vi "from string.vi"(8 "error in":errorcluster, 9 "data":string, 10 "version":string, 11 "Engine configuration in":refnum<class "Engine configuration.lvclass">) -> (0 "error out":errorcluster, 3 "Engine configuration out":refnum<class "Engine configuration.lvclass">)   [LabVIEW 2025, in "Abstract Engine.lvlib" / "Engine configuration.lvclass"]
doc: "Provides an interface for loading a module configuration from a file or other serialized data source. It is recommended that all children of this class store data in two sets--data required for its own initialization, and any data required for parent initialization--and that each implementation uses the <b>Call Parent Method</b> primitive to de-serialize parent information.Copyright 2017 National Instruments Corporation\n\nLicensed under the Apache License, Version 2.0 (the \"License\"); you may not use this file except in compliance with the License. You may obtain a copy of the License at http://www.apache.org/licenses/LICENSE-2.0\nUnless required by applicable law or agreed to in writing, software distributed under the License is distributed on an \"AS IS\" BASIS, WITHOUT WARRANTIES OR CONDITIONS OF ANY KIND, either express or implied. See the License for the specific language governing permissions and limitations under the License."
uses:
  Engine configuration.lvclass
  Engine configuration.lvclass/Engine configuration.ctl
  Engine Setting.ctl
  Users/Public/Documents/Sandia National Labs/TSS Plugin/CEF.lvlibp/serializable configuration/CEF_serializable configuration.lvclass
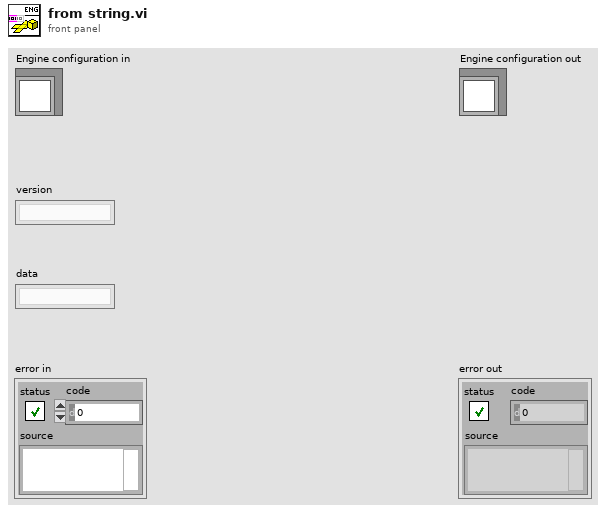
[diagram p1: front panel]
types:
  T1 = typedef "Abstract Engine.lvlib/Engine configuration.lvclass/Engine Setting.ctl" = cluster{"Enabled":bool, "IP Address":string, "Port":i32, "Description":string, "Type":string, "Version":string}
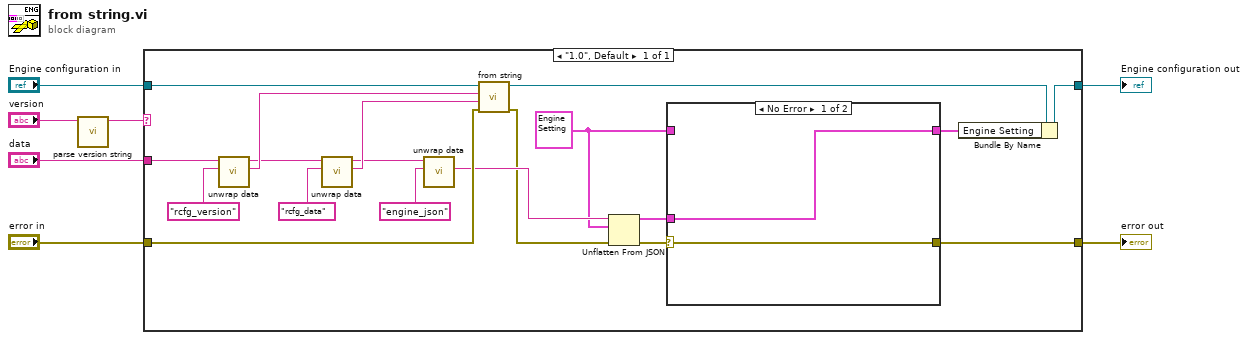
[diagram p0: block diagram]
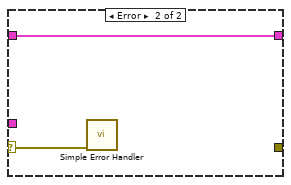
[diagram p2: hidden frame]
diagram:
  n1 = call "parse version string.vi"("full version"="version") -> ("major.minor version"=w1:string)  [unwired: 7 in, 3 out]
  n2 = case shown="\"1.0\", Default" w1 {
    tunnel: "Engine configuration in" -> [w26]
    tunnel: [w15] -> w6
    tunnel: "data" -> [w24]
    tunnel: "error in" -> [w16]
    tunnel: [w8] -> w5
    frame "1.0", Default {
      w9 = T1 {"Enabled"=TRUE, "IP Address"="", "Port"=0, "Description"="Type = Class \n", "Type"="none", "Version"="none"} ("Default Engine")
      n3 = call "unwrap data.vi"("identifier"="rcfg_version" ("additional identifier"), "data to unwrap"=w24) -> ("unwrapped data"=w22:string, "remaining string"=w21:string)  [unwired: 8 in]
      n4 = call "unwrap data.vi"("identifier"="rcfg_data" ("additional identifier"), "data to unwrap"=w21) -> ("unwrapped data"=w19:string, "remaining string"=w18:string)  [unwired: 8 in]
      n5 = call "unwrap data.vi"("identifier"="engine_json" ("additional identifier"), "data to unwrap"=w18) -> ("unwrapped data"=w14:string)  [unwired: 8 in, 1 out]
      n6 = call-parent "from string.vi"("error in"=w16, "data"=w19, "version"=w22, "CEF_Configuration in"=w26) -> ("error out"=w13:errorcluster, "CEF_Configuration out"=w25:refnum<class "Engine configuration.lvclass">)  [unwired: 6 in]
      n7 = Unflatten From JSON(JSON string=w14, type and defaults=w9, error in (no error)=w13) -> (value=w11:T1, error out=w12:errorcluster)  [unwired: 4 in]
      n8 = case shown="No Error" w12 {
        selector: w12 -> [w27 w29]
        tunnel: w11 -> [w28 _]
        tunnel: [w28 w30] -> w10
        tunnel: w9 -> [_ w30]
        tunnel: [w27 _] -> w8
        frame No Error {
        }
        frame Error {
          n9 = call <vilib>:"Simple Error Handler.vi"("error in (no error)"=w29) -> ()  [unwired: 4 in, 5 out]
        }
      }
      n10 = Bundle By Name(cluster=w25, "Engine Setting"=w10) -> (w15:refnum<class "Engine configuration.lvclass">)
    }
  }
  "error out" <- w5
  "Engine configuration out" <- w6
